vi "Agilent PWM Set Stimulus.vi"(7 "Agilent PWM":T2, 8 "error in (no error)":errorcluster, 10 "Stimulus":T1, 11 "VISA Resource Name":refnum<visa-resource-name>) -> (0 "error out":errorcluster {"code" format="%.0x"}, 3 "dup VISA Resource Name":refnum<visa-resource-name>)   [LabVIEW 2011]
uses:
  TypeDefs/Agilent PWM Instrument Info.ctl
  PWM Parameters.ctl
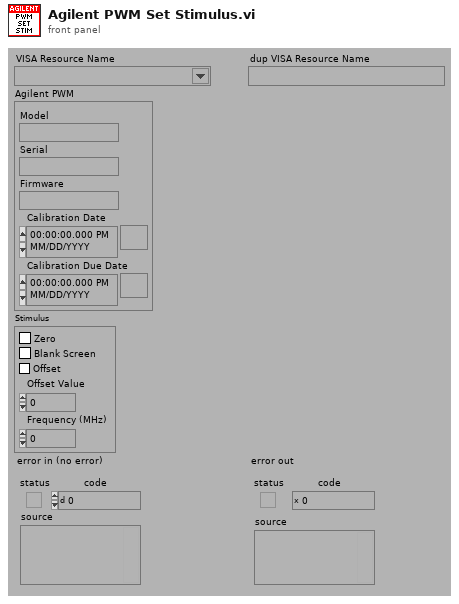
[diagram p1: front panel]
types:
  T1 = typedef "PWM Parameters.ctl" = cluster{"Zero":bool, "Blank Screen":bool, "Offset":bool, "Offset Value":dbl, "Frequency (MHz)":dbl}
  T2 = typedef "Agilent PWM Instrument Info.ctl" = cluster{"Model":string, "Serial":string, "Firmware":string, "Calibration Date":timestamp, "Calibration Due Date":timestamp}
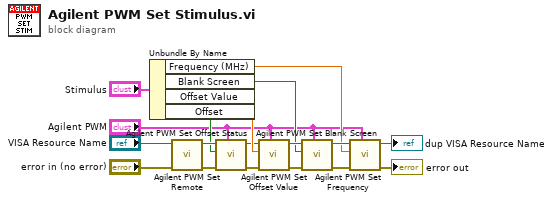
[diagram p0: block diagram]
diagram:
  n1 = Unbundle By Name("Stimulus") -> ("Frequency (MHz)"=w2:dbl, "Blank Screen"=w7:bool, "Offset Value"=w12:dbl, "Offset"=w13:bool)
  n2 = call "Agilent PWM Set Remote.vi"("error in (no error)"="error in (no error)", "VISA Resource Name"="VISA Resource Name") -> ("error out"=w17:errorcluster, "dup VISA Resource Name"=w16:refnum<visa-resource-name>)  [unwired: 8 out]
  n3 = call "Agilent PWM Set Offset Status.vi"("Agilent PWM"="Agilent PWM", "error in (no error)"=w17, "On/Off"=w13, "VISA Resource Name"=w16) -> ("error out"=w10:errorcluster, "dup VISA Resource Name"=w11:refnum<visa-resource-name>)  [unwired: 6 out]
  n4 = call "Agilent PWM Set Offset Value.vi"("Agilent PWM"="Agilent PWM", "error in (no error)"=w10, "Offset Value (dBm)"=w12, "VISA Resource Name"=w11) -> ("error out"=w9:errorcluster, "dup VISA Resource Name"=w8:refnum<visa-resource-name>)  [unwired: 1 in, 5 out]
  n5 = call "Agilent PWM Set Blank Screen.vi"("Agilent PWM"="Agilent PWM", "error in (no error)"=w9, "Blank Screen"=w7, "VISA Resource Name"=w8) -> ("error out"=w6:errorcluster, "dup VISA Resource Name"=w5:refnum<visa-resource-name>)  [unwired: 6 out]
  n6 = call "Agilent PWM Set Frequency.vi"("Agilent PWM"="Agilent PWM", "error in (no error)"=w6, "Frequency (MHz)"=w2, "VISA Resource Name"=w5) -> ("error out"=→"error out":errorcluster, "dup VISA Resource Name"=→"dup VISA Resource Name":refnum<visa-resource-name>)  [unwired: 6 in]
